vi "LatestAPLPath.vi"(8 "Error In":errorcluster, 9 "APL Search String":T1(ring), 11 "Folder Path":path=path "\\\\itnas.appl.ge.com\\technology/Electronics/InProcess/Software/ci_builds/2015_VA_Washer") -> (0 "Error Out":errorcluster, 1 "Report text":string, 2 "Found ?":bool, 3 "File Path":path=path "\\\\itnas.appl.ge.com\\technology/Electronics/InProcess/Software/ci_builds/2015_VA_Washer/2015-03-06_03-42-38(Build-1952)/Binaries/2015VAWasher_Param_QA_Cycle_1_62_99_1.apl")   [LabVIEW 2016, in "2015 VA Washer.lvlib"]
doc: "This VI will search for the most recent version of software apls and return its path. You can search for various firware or xml apls.\n\nIf not found it will return an empty path, as well and boolean and report text."
uses:
  Projects/2015 VA Washer.lvlib
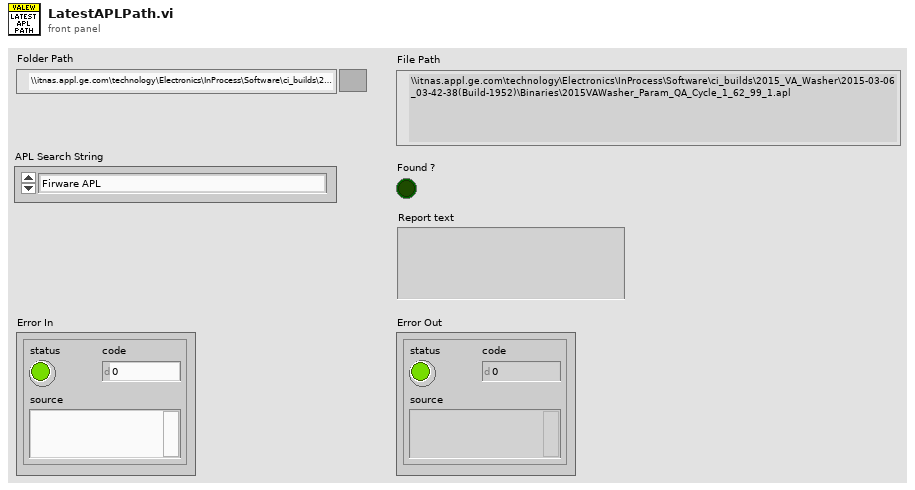
[diagram p1: front panel]
types:
  T1 = enum16{"Firware APL", "QA XML APL", "System XML", "QA Cycle XML APL", "Reliability Cycle XML", "ERD Definitions XML"}
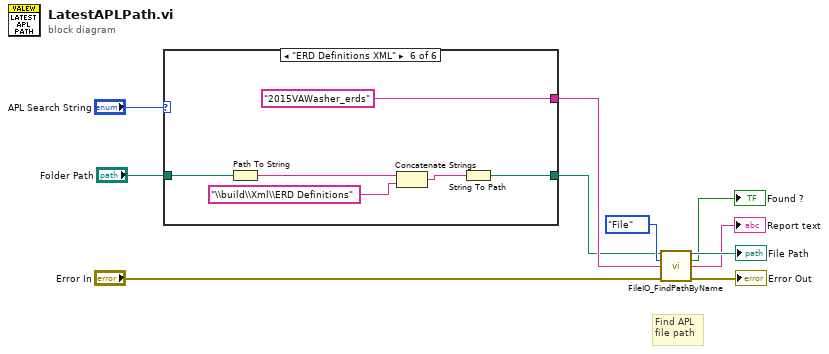
[diagram p0: block diagram]
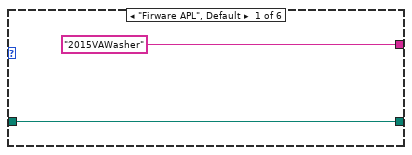
[diagram p2: hidden frame]
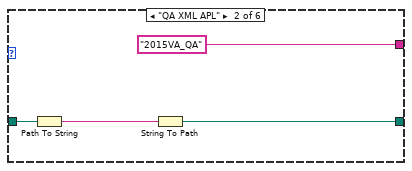
[diagram p3: hidden frame]
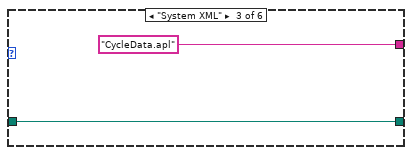
[diagram p4: hidden frame]
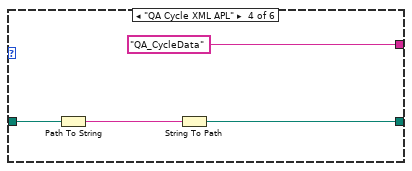
[diagram p5: hidden frame]
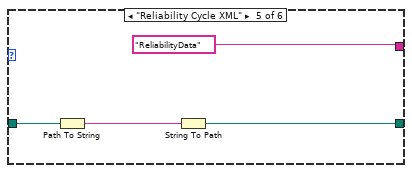
[diagram p6: hidden frame]
diagram:
  # "Find APL\nfile path"
  n1 = case shown="\"ERD Definitions XML\"" "APL Search String" {
    tunnel: ["2015VAWasher" "2015VA_QA" "CycleData.apl" "QA_CycleData" "ReliabilityData" "2015VAWasher_erds"] -> w7
    tunnel: [w11 w13 w17 w19 w23 w27] -> w1
    tunnel: "Folder Path" -> [w11 w14 w17 w20 w24 w28]
    frame "Firware APL", Default {
    }
    frame "QA XML APL" {
      n2 = Path To String(path=w14) -> (string=w15:string)
      n3 = String To Path(string=w15) -> (path=w13:path)
    }
    frame "System XML" {
    }
    frame "QA Cycle XML APL" {
      n4 = Path To String(path=w20) -> (string=w21:string)
      n5 = String To Path(string=w21) -> (path=w19:path)
    }
    frame "Reliability Cycle XML" {
      n6 = Path To String(path=w24) -> (string=w25:string)
      n7 = String To Path(string=w25) -> (path=w23:path)
    }
    frame "ERD Definitions XML" {
      n8 = Path To String(path=w28) -> (string=w32:string)
      n9 = Concatenate Strings(w32, "\\build\\Xml\\ERD Definitions" ("string")) -> (w30:string)
      n10 = String To Path(string=w30) -> (path=w27:path)
    }
  }
  n11 = call "FileIO_FindPathByName.vi"("Path In"=w1, "File or Folder ?"=enum16{"Folder", "File"}."File", "File/Folder Search String"=w7, "Error In"="Error In") -> ("Path Out"=→"File Path":path, "Found ?"=→"Found ?":bool, "Report Text"=→"Report text":string, "Error Out"=→"Error Out":errorcluster)  [unwired: 8 in]
